vi "Settings Dialog.vi"(0 "Settings in":T9 {"Processing Settings"."Test Parameters"."Allowed Tolerance (%) FS" format="%#_4g"; "Acq Settings"."Config Settings"."Simulated Sensor Injection" scale=0.0..100.0}, 1 "Database in":refnum<queue>, 11 "error in (no error)":errorcluster) -> (3 "Database out":refnum<queue>, 4 "Settings out":T9 {"Processing Settings"."Test Parameters"."Allowed Tolerance (%) FS" format="%#_4g"; "Acq Settings"."Config Settings"."Simulated Sensor Injection" scale=0.0..100.0}, 6 "Measurements out":T7[](array[typedef]), 8 "UI Refresh Needed?":bool, 10 "Cancelled?":bool, 15 "error out":errorcluster)   [LabVIEW 2026, in "Settings.lvlib"]
doc: "Dialog for selecting user specified settings."
uses:
  Settings.lvlib
  controls/UI/Settings Cluster.ctl
  controls/UI/Acq Settings.ctl
  Acquisition/Instrument Specifications Configuration.ctl
  Acquisition/Instrument Specifications Cluster Configuration.ctl
  controls/UI/Measurement Role.ctl
  controls/UI/Config Settings.ctl
  Processing/Processing Settings.ctl
  controls/Messaging Payloads/Sensor CoreData.ctl
  controls/Messaging Payloads/Sensor CoreData Cluster.ctl
  controls/UI/Units Enum.ctl
  controls/UI/Signal Enum.ctl
  Processing/Test Parameters.ctl
  Processing/Test Parameters Cluster.ctl
  controls/UI/Test Sequence Context.ctl
  controls/UI/Direction.ctl
  controls/UI/Session Identfiers.ctl
  controls/UI/Test Sequence Settings.ctl
  controls/UI/Test Sequence State.ctl
  controls/UI/Test Sequence Enum.ctl
  controls/Controller/Stimulus Settings.ctl
  controls/Controller/Stimulus Outputs.ctl
  controls/Controller/Stimulus Output.ctl
  controls/Controller/Controller Core Data.ctl
  controls/Controller/Stimulus Output Configuration.ctl
  controls/Controller/Stimulus Role.ctl
  support/Architecture/Message Queue/Message Cluster.ctl
  controls/UI/Measurements Config.ctl
  controls/UI/Measurement Config.ctl
  controls/UI/Stimulus Outputs Display.ctl
  controls/UI/Stimulus Output Display.ctl
  controls/UI/Settings Refs.ctl
  controls/UI/UI List Type.ctl
  controls/UI/Data Entity.ctl
  controls/UI/Measurement Role Selection.ctl
  Acquisition/Acquisition.lvlib
  support/Architecture/Message Queue/Message Queue.lvlib
  Processing/Processing_Engine.lvlib
panel:
  in  "STIMULUS OUTPUTS":T1
  out "INSTRUMENT CONFIGURATIONS":T4
  in  "MEASUREMENTS":T8
  in  "Operator":string(combo)
  in  "Cancel Button":bool
  in  "OK Button":bool
  # "Non visible portion of dialog (needed for connector pane)."
  # "* Database-configured values. Maintained by an Administrator."
  # "Physical Channel and Measurement Role are assigned in the Measurements section."
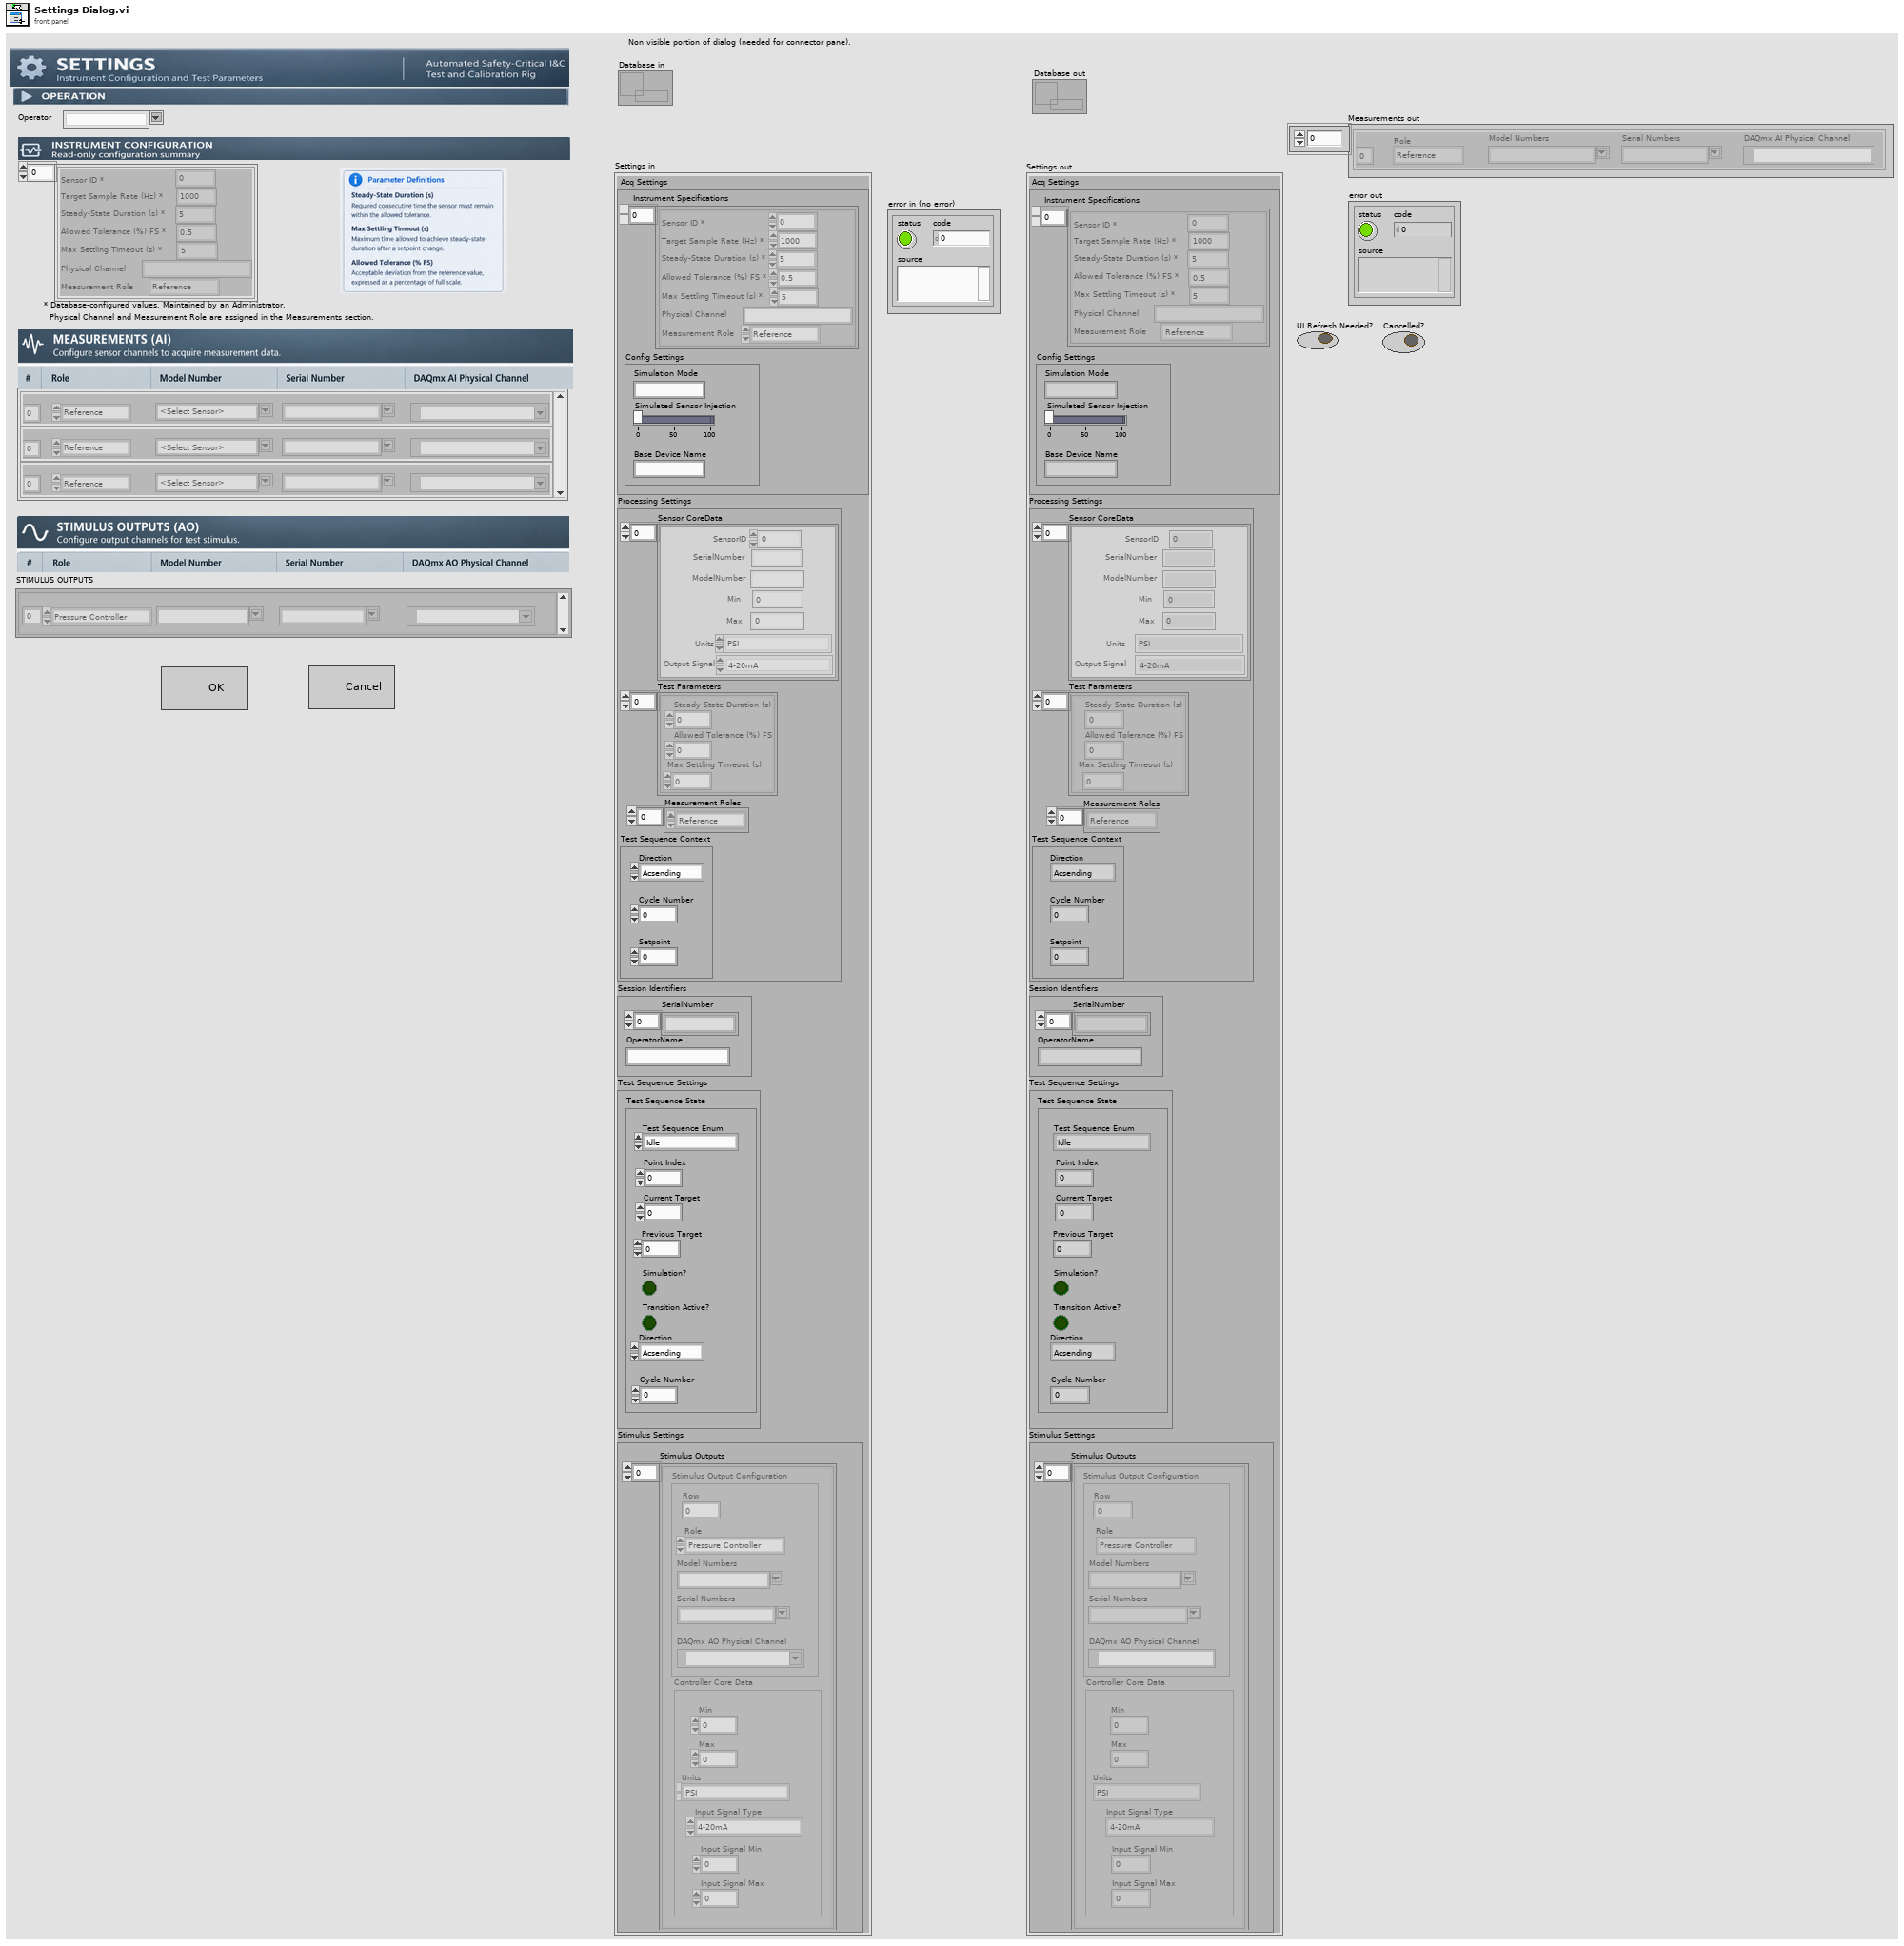
[diagram p1: front panel]
types:
  T1 = typedef "Settings.lvlib/Stimulus Outputs Display.ctl" = T2[]
  T2 = typedef "Settings.lvlib/Stimulus Output Display.ctl" = cluster{"DAQmx AO Physical Channel":tag, "Role":T3, "Model Numbers":string, "Serial Numbers":string, "Row":i32}
  T3 = typedef "Stimulus Role.ctl" = enum16{"Pressure Controller", "Temperature Controller"}
  T4 = typedef "Acquisition.lvlib/Instrument Specifications Configuration.ctl" = T5[]
  T5 = typedef "Acquisition.lvlib/Instrument Specifications Cluster Configuration.ctl" = cluster{"Sensor ID *":i32, "Target Sample Rate (Hz) *":dbl, "Steady-State Duration (s) *":i32, "Allowed Tolerance (%) FS *":dbl, "Max Settling Timeout (s) *":i32, "Physical Channel":string, "Measurement Role":T6}
  T6 = typedef "Settings.lvlib/Measurement Role.ctl" = enum16{"Reference", "UUT"}
  T7 = typedef "Measurement Config.ctl" = cluster{"DAQmx AI Physical Channel":tag, "Serial Numbers":string, "Model Numbers":string, "Role":T6, "Row":i32}
  T8 = typedef "Measurements Config.ctl" = T7[]
  T9 = typedef "Settings Cluster.ctl" = cluster{"Acq Settings":T10, "Processing Settings":T12, "Session Identifiers":T21, "Test Sequence Settings":T22, "Stimulus Settings":T25}
  T10 = typedef "Acq Settings.ctl" = cluster{"Instrument Specifications":T4, "Config Settings":T11}
  T11 = typedef "Config Settings.ctl" = cluster{"Simulated Sensor Injection":dbl, "Base Device Name":string, "Simulation Mode":string}
  T12 = typedef "Processing_Engine.lvlib/Processing Settings.ctl" = cluster{"Sensor CoreData":T13, "Test Parameters":T17, "Measurement Roles":T6[], "Test Sequence Context":T19}
  T13 = typedef "Sensor CoreData.ctl" = T14[]
  T14 = typedef "Settings.lvlib/Sensor CoreData Cluster.ctl" = cluster{"SerialNumber":string, "ModelNumber":string, "Min":dbl, "Max":dbl, "Units":T15, "Output Signal":T16, "SensorID":i32}
  T15 = typedef "Units Enum.ctl" = enum16{"PSI", "Deg C", "kPa", "GPM"}
  T16 = typedef "Signal Enum.ctl" = enum16{"4-20mA", "0-10V", "Thermocouple Type K"}
  T17 = typedef "Processing_Engine.lvlib/Test Parameters.ctl" = T18[]
  T18 = typedef "Settings.lvlib/Test Parameters Cluster.ctl" = cluster{"Steady-State Duration (s)":i32, "Allowed Tolerance (%) FS":dbl, "Max Settling Timeout (s)":i32}
  T19 = typedef "Settings.lvlib/Test Sequence Context.ctl" = cluster{"Direction":T20, "Cycle Number":i32, "Setpoint":dbl}
  T20 = typedef "Settings.lvlib/Direction.ctl" = enum16{"Acsending", "Descending"}
  T21 = typedef "Session Identfiers.ctl" = cluster{"SerialNumber":string[], "OperatorName":string}
  T22 = typedef "Test Sequence Settings.ctl" = cluster{"Test Sequence State":T23}
  T23 = typedef "Settings.lvlib/Test Sequence State.ctl" = cluster{"Test Sequence Enum":T24, "Point Index":i32, "Current Target":dbl, "Previous Target":dbl, "Simulation?":bool, "Direction":T20, "Transition Active?":bool, "Cycle Number":i32}
  T24 = typedef "Test Sequence Enum.ctl" = enum16{"Idle", "Start Point", "Point Complete", "Test Complete", "Abort Test", "Reset"}
  T25 = typedef "Settings.lvlib/Stimulus Settings.ctl" = cluster{"Stimulus Outputs":T26}
  T26 = typedef "Settings.lvlib/Stimulus Outputs.ctl" = T27[]
  T27 = typedef "Settings.lvlib/Stimulus Output.ctl" = cluster{"Controller Core Data":T28, "Stimulus Output Configuration":T29}
  T28 = typedef "Settings.lvlib/Controller Core Data.ctl" = cluster{"Min":dbl, "Max":dbl, "Units":T15, "Input Signal Type":T16, "Input Signal Min":dbl, "Input Signal Max":dbl}
  T29 = typedef "Settings.lvlib/Stimulus Output Configuration.ctl" = cluster{"DAQmx AO Physical Channel":tag, "Role":T3, "Model Numbers":string, "Serial Numbers":string, "Row":i32}
  T30 = typedef "Settings Refs.ctl" = cluster{"Serial Numbers Ref":refnum<vi>, "Logging Ref":refnum<vi>, "Model Numbers Ref":refnum<vi>, "OK Ref":refnum<vi>, "Instrument Specifications Cluster Ref":refnum<vi>, "Instrument Specifications Ref":refnum<vi>, "Measurements Ref":refnum<vi>, "Stimulus Outputs Ref":refnum<vi>}
  T31 = typedef "Settings.lvlib/Measurement Role Selection.ctl" = enum16{"Controller", "Reference", "UUT", "All"}
  T32 = typedef "Settings.lvlib/Data Entity.ctl" = enum16{"Measurement", "Controller", " Test Configuration"}
  T33 = enum8{"Enabled", "Disabled", "Disabled and Grayed Out"}
  T34 = typedef "UI List Type.ctl" = enum16{"Model Numbers", "Serial Numbers", "Operators", "Calibration Points", "Start Run Times"}
  T35 = typedef "LVPoint32TypeDef.ctl" = cluster{"Horizontal":i32, "Vertical":i32}
  T36 = typedef "MSG FetchConfiguration Payload.ctl" = cluster{"Serial Numbers":string[], "Hardware Settings Cluster":T5}
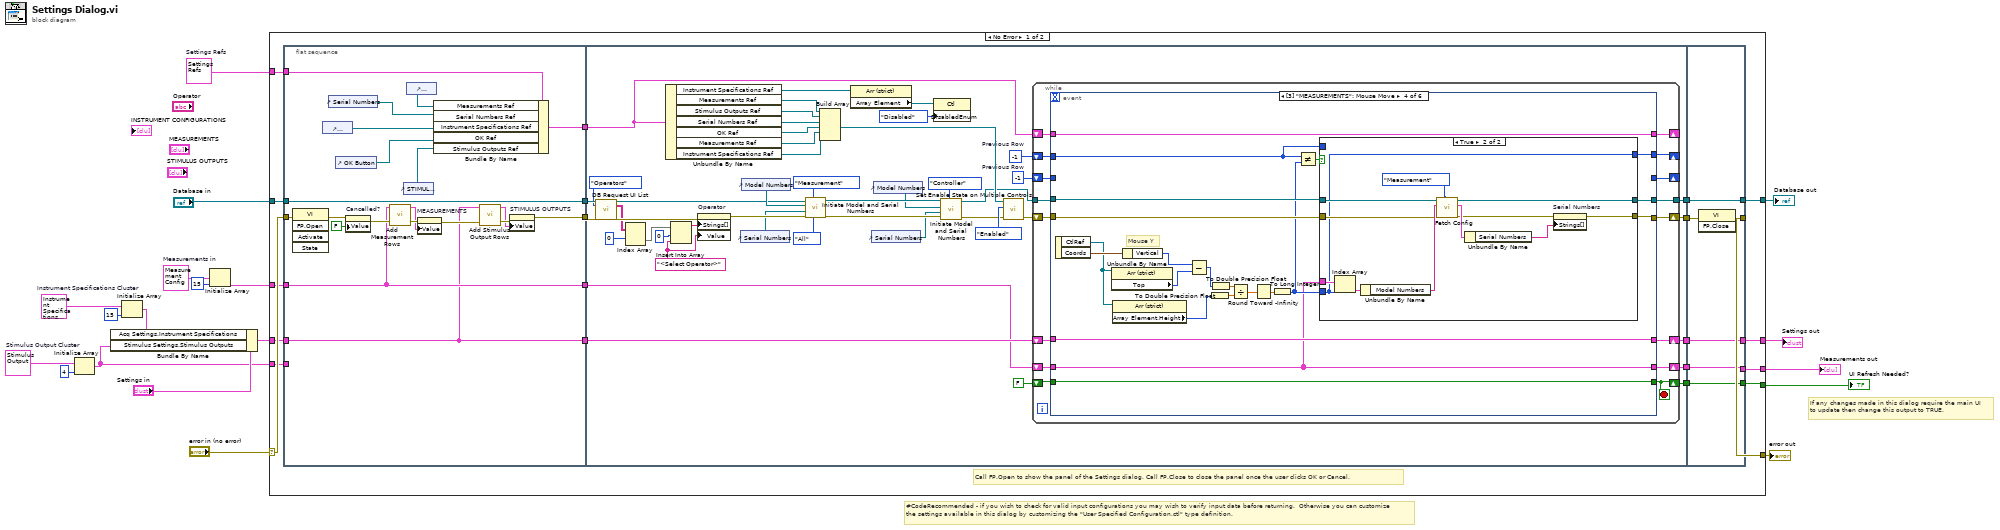
[diagram p0: block diagram]
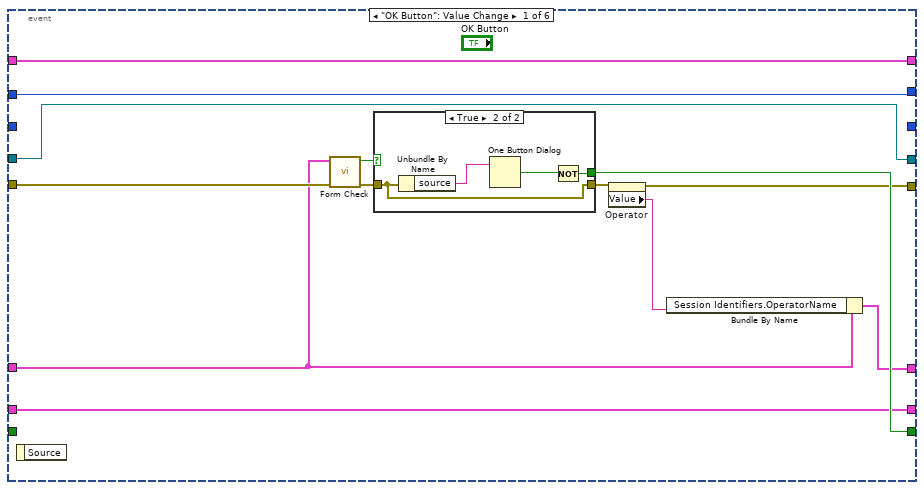
[diagram p2: hidden frame]
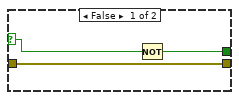
[diagram p3: hidden frame]
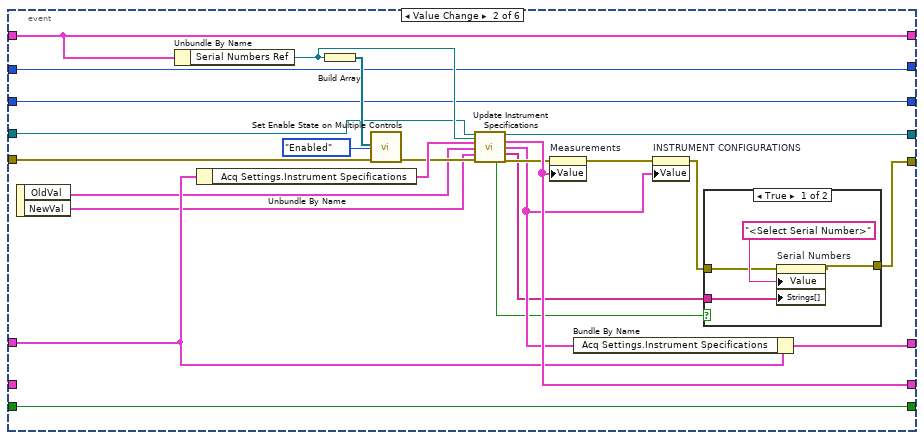
[diagram p4: hidden frame]
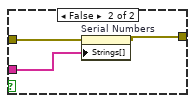
[diagram p5: hidden frame]
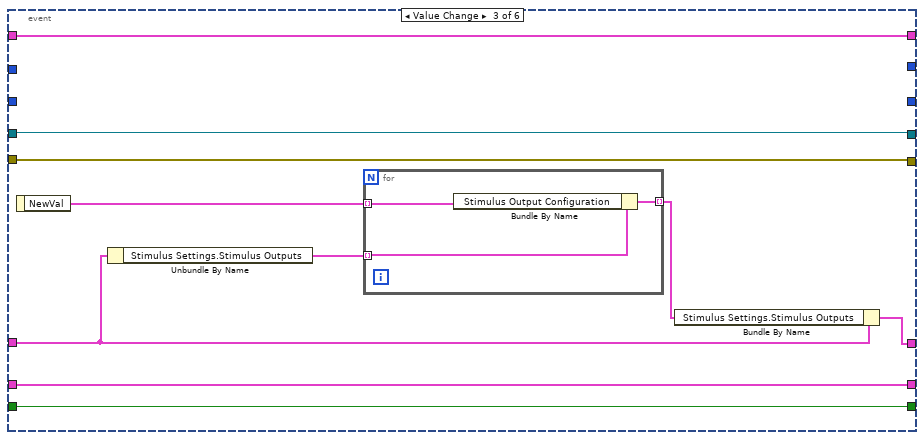
[diagram p6: hidden frame]
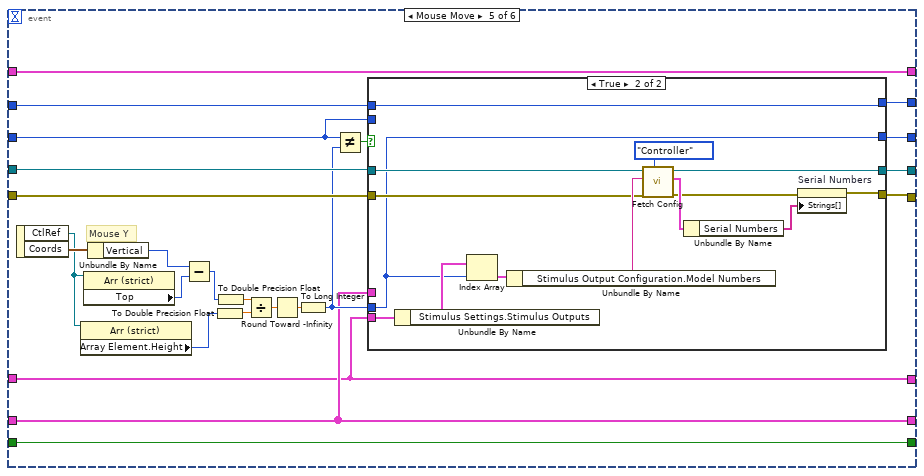
[diagram p8: hidden frame]
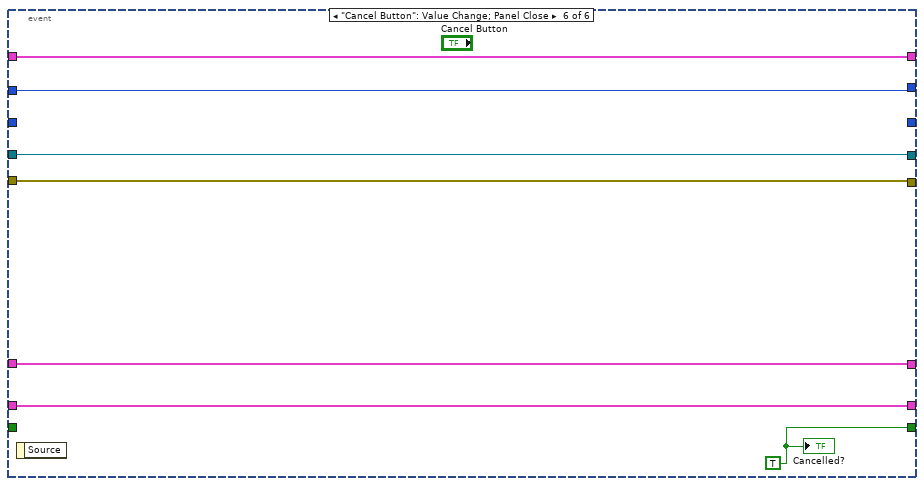
[diagram p10: hidden frame]
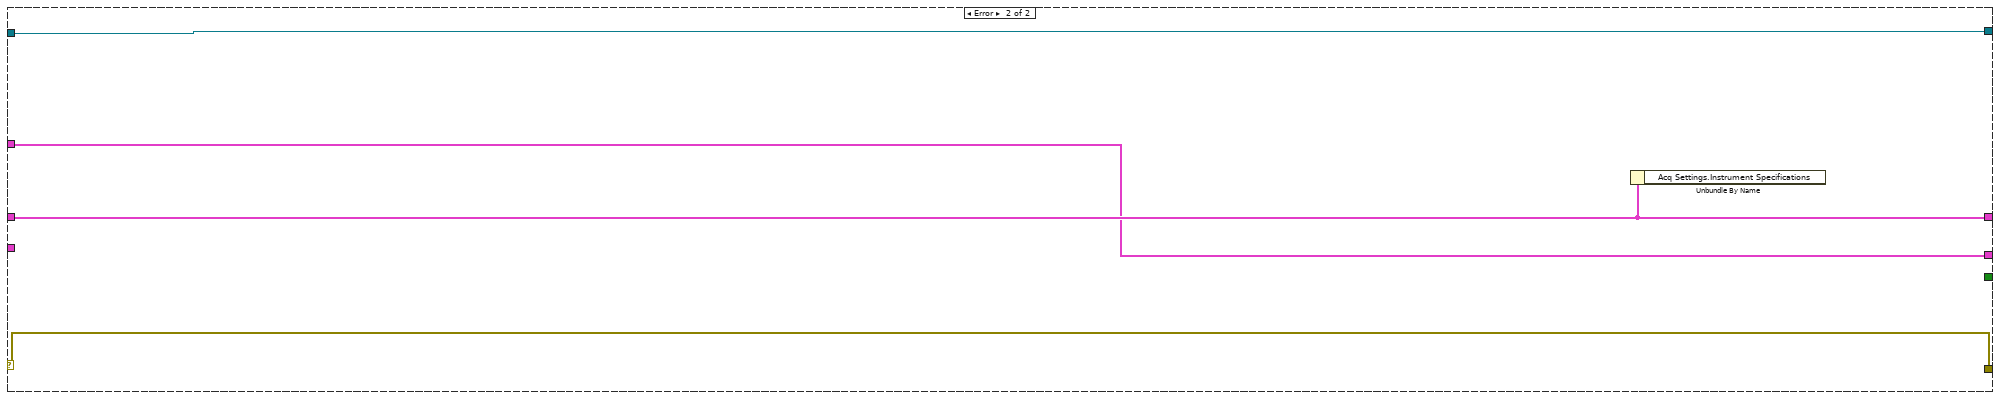
[diagram p11: hidden frame]
diagram:
  w2 = T27 {"Controller Core Data"={"Min"=0.0, "Max"=0.0, "Units"=enum."PSI", "Input Signal Type"=enum."4-20mA", "Input Signal Min"=0.0, "Input Signal Max"=0.0}, "Stimulus Output Configuration"={"DAQmx AO Physical Channel"="", "Role"=enum."Pressure Controller", "Model Numbers"="", "Serial Numbers"="", "Row"=0}}  # Stimulus Output Cluster
  w8 = T5 {"Sensor ID *"=0, "Target Sample Rate (Hz) *"=1000.0, "Steady-State Duration (s) *"=5, "Allowed Tolerance (%) FS *"=0.5, "Max Settling Timeout (s) *"=5, "Physical Channel"="", "Measurement Role"=enum."Reference"}  # Instrument Specifications Cluster
  w12 = T7 {"DAQmx AI Physical Channel"="", "Serial Numbers"="", "Model Numbers"="<Select Sensor>", "Role"=enum."Reference", "Row"=0}  # Measurements in
  w16 = T30 {"Serial Numbers Ref"=refnum, "Logging Ref"=refnum, "Model Numbers Ref"=refnum, "OK Ref"=refnum, "Instrument Specifications Cluster Ref"=refnum, "Instrument Specifications Ref"=refnum, "Measurements Ref"=refnum, "Stimulus Outputs Ref"=refnum}  # Settings Refs
  # "If any changes made in this dialog require the main UI to update then change this output to TRUE."
  # "#CodeRecommended - if you wish to check for valid input configurations you may wish to verify input data before returning.  Otherwise you can customize the settings available in this dialog by customizing the \"User Specified Configuration.ctl\" type definition."
  n1 = Initialize Array(w2, 4 ("dimension size")) -> (w1:T27[])
  n2 = Initialize Array(w8, 15 ("dimension size")) -> (w7:T5[])
  n3 = Bundle By Name(cluster="Settings in", "Acq Settings.Instrument Specifications"=w7, "Stimulus Settings.Stimulus Outputs"=w1) -> (w6:T9)
  n4 = Initialize Array(w12, 15 ("dimension size")) -> (w10:T7[])
  n5 = case shown="No Error" "error in (no error)" {
    selector: "error in (no error)" -> [w32 w282]
    tunnel: [w36 w282] -> w18
    tunnel: [w27 _] -> w17
    tunnel: "Database in" -> [w38 w280]
    tunnel: w16 -> [w33 _]
    tunnel: [w28 w281] -> w15
    tunnel: w6 -> [w30 w281]
    tunnel: [w25 w280] -> w14
    tunnel: w10 -> [w24 w279]
    tunnel: [w21 w279] -> w13
    tunnel: w1 -> [w20 _]
    frame No Error {
      # "Call FP.Open to show the panel of the Settings dialog. Call FP.Close to close the panel once the user clicks OK or Cancel."
      n6 = flat-sequence {
        tunnel: w38 -> [w59]
        tunnel: [w44] -> w35
        tunnel: w32 -> [w60]
        tunnel: [w59] -> w34
        tunnel: w33 -> [w56]
        tunnel: [w58] -> w31
        tunnel: w30 -> [w41]
        tunnel: [w41] -> w29
        tunnel: w24 -> [w42]
        tunnel: [w42] -> w23
        tunnel: w20 -> [_]
        tunnel: [w106] -> w40
        tunnel: [w105] -> w39
        tunnel: w35 -> [w98]
        tunnel: [w104] -> w37
        tunnel: w34 -> [w99]
        tunnel: w31 -> [w101]
        tunnel: w29 -> [w100]
        tunnel: [w92] -> w26
        tunnel: w23 -> [w88]
        tunnel: [w91] -> w22
        tunnel: [w278] -> w28
        tunnel: w40 -> [w275]
        tunnel: w39 -> [w278]
        tunnel: w37 -> [w277]
        tunnel: [w276] -> w36
        tunnel: [w275] -> w27
        tunnel: w26 -> [w274]
        tunnel: [w274] -> w25
        tunnel: w22 -> [w273]
        tunnel: [w273] -> w21
        frame #0 {
          n7 = invoke class="VI" method="FP.Open"(error in=w60) -> (error out=w55:errorcluster)  [unwired: 4 in, 4 out]
          n8 = control-ref of="INSTRUMENT CONFIGURATIONS"() -> (w50:refnum<vi>)
          n9 = control-ref of="Serial Numbers"() -> (w53:refnum<vi>)
          n10 = control-ref of="OK Button"() -> (w57:refnum<vi>)
          n11 = property on="Cancelled?" class="Bool (strict)"(error in=w55, "Value"=FALSE ("Cancelled?")) -> (error out=w49:errorcluster)  [unwired: 1 in, 1 out]
          n12 = call "Add Measurement Rows.vi"("error in (no error)"=w49, "Measurements in"=w42) -> ("error out"=w48:errorcluster, "Measurements out"=w47:T8)  [unwired: 8 in]
          n13 = control-ref of="STIMULUS OUTPUTS"() -> (w51:refnum<vi>)
          n14 = control-ref of="MEASUREMENTS"() -> (w52:refnum<vi>)
          n15 = property on="MEASUREMENTS" class="Arr (strict)"(error in=w48, "Value"=w47) -> (error out=w46:errorcluster)  [unwired: 1 in, 1 out]
          n16 = Bundle By Name(cluster=w56, "Measurements Ref"=w52, "Serial Numbers Ref"=w53, "Instrument Specifications Ref"=w50, "OK Ref"=w57, "Stimulus Outputs Ref"=w51) -> (w58:T30)
          n17 = call "Add Stimulus Output Rows.vi"("error in (no error)"=w46, "Settings"=w41) -> ("error out"=w45:errorcluster, "Stimulus Outputs"=w43:T1)  [unwired: 8 in]
          n18 = property on="STIMULUS OUTPUTS" class="Arr (strict)"(error in=w45, "Value"=w43) -> (error out=w44:errorcluster)  [unwired: 1 in, 1 out]
        }
        frame #1 {
          w65 = -1  # Previous Row
          w89 = -1  # Previous Row
          w93 = "<Select Operator>"
          n19 = call "DB Request UI List.vi"("Database in"=w99, "UI List Type"=UI_List_Type."Operators", "error in (no error)"=w98) -> ("Database out"=w75:refnum<queue>, "Results"=w64:string[][], "error out"=w95:errorcluster)  [unwired: 14 in]
          n20 = Index Array(array=w64, index (row)=0 ("index")) -> (element=w62:string[])  [unwired: 1 in]
          n21 = Unbundle By Name(w101) -> ("Instrument Specifications Ref"=w80:refnum<vi>, "Measurements Ref"=w84:refnum<vi>, "Stimulus Outputs Ref"=w86:refnum<vi>, "Serial Numbers Ref"=w85:refnum<vi>, "OK Ref"=w82:refnum<vi>, "Measurements Ref"=w83:refnum<vi>, "Instrument Specifications Ref"=w81:refnum<vi>)
          n22 = Insert Into Array(array=w62, index=0, new element=w93) -> (w96:string[])
          n23 = property on="Operator" class="CmbBox"(error in=w95, "Strings[]"=w96, "Value"=w93) -> (error out=w94:errorcluster)  [unwired: 1 in, 1 out]
          n24 = control-ref of="Serial Numbers"() -> (w74:refnum<vi>)
          n25 = control-ref of="Model Numbers"() -> (w76:refnum<vi>)
          n26 = call "Initiate Model and Serial Numbers.vi"("Measurement Role Selection"=Measurement_Role_Selection."All" ("Measurement Role"), "UI Device Type"=Data_Entity."Measurement", "error in (no error)"=w94, "Serial CmbBox Ref"=w74, "Model CmbBox Ref"=w76, "Database in"=w75) -> ("error out"=w73:errorcluster, "Database out"=w71:refnum<queue>)  [unwired: 4 in]
          n27 = Build Array(w84, w86, w85, w82, w83, w81) -> (w102:refnum<vi>[])
          n28 = property class="Arr (strict)"(reference=w80) -> ("Array Element"=w79:refnum<vi>)  [unwired: 1 in, 2 out]
          n29 = control-ref of="Serial Numbers"() -> (w66:refnum<vi>)
          n30 = control-ref of="Model Numbers"() -> (w67:refnum<vi>)
          n31 = property class="Ctl"(reference=w79, "DisabledEnum"=T33."Disabled" ("Disabled")) -> ()  [unwired: 1 in, 2 out]
          n32 = call "Initiate Model and Serial Numbers.vi"("UI Device Type"=Data_Entity."Controller", "error in (no error)"=w73, "Serial CmbBox Ref"=w66, "Model CmbBox Ref"=w67, "Database in"=w71) -> ("error out"=w72:errorcluster, "Database out"=w70:refnum<queue>)  [unwired: 5 in]
          n33 = call "Set Enable State on Multiple Controls.vi"("Controls"=w102, "Disabled"=T33."Enabled", "error in (no error)"=w72) -> ("error out"=w77:errorcluster)  [unwired: 7 in]
          n34 = while {
            tunnel: w70 -> [w118]
            shift-right: [w122] -> w105
            shift-left: w100 -> [w121]
            shift-right: [w120] -> w104
            shift-left: w77 -> [w119]
            shift-right: [w114] -> w106
            shift-left: FALSE ("UI Refresh Needed?") -> [w117]
            shift-right: [w115] -> _
            shift-left: w101 -> [w116]
            tunnel: [w113] -> w92
            shift-right: [w109] -> _
            shift-left: w89 -> [w110]
            shift-right: [w112] -> w91
            shift-left: w88 -> [w111]
            shift-right: [w107] -> _
            shift-left: w65 -> [w108]
            stop <- w114 stop-if-true
            n35 = event shown="[3] \"MEASUREMENTS\": Mouse Move" {
              selector: _ -> [_ _ _ _ _ _]
              dyn-events: _ -> [_ _ _ _ _ _]
              timeout: _ -> [_ _ _ _ _ _]
              tunnel: [w128 w160 w178 w208 w225 w272] -> w122
              tunnel: w121 -> [w125 w161 w180 w208 w225 w272]
              tunnel: [w132 w166 w176 w187 w228 w270] -> w114
              tunnel: w119 -> [w134 w159 w175 w195 w235 w271]
              tunnel: [w126 w150 w175 w189 w230 w271] -> w120
              tunnel: w118 -> [w127 w145 w182 w196 w236 w268]
              tunnel: w117 -> [_ w166 w176 w187 w228 _]
              tunnel: w116 -> [w131 w147 w183 w207 w247 w269]
              tunnel: [w131 w147 w183 w207 w247 w269] -> w115
              tunnel: [w127 w144 w182 w194 w234 w268] -> w113
              tunnel: [w124 w165 w177 w188 w229 w267] -> w112
              tunnel: w111 -> [w124 _ w177 w188 w229 w267]
              tunnel: w110 -> [w123 w148 _ w190 w231 w266]
              tunnel: [w123 w148 _ w191 w232 w266] -> w109
              tunnel: w108 -> [_ w143 _ _ w226 _]
              tunnel: [_ w143 _ _ w224 _] -> w107
              event "OK Button": Value Change {
                n36 = event-data() -> ()  [unwired: 1 in, 1 out]
                n37 = call "Form Check.vi"("error in (no error)"=w134, "Config in"=w125) -> ("error out"=w133:errorcluster, "Form Error?"=w135:bool)  [unwired: 8 in]
                n38 = case shown="True" w135 {
                  selector: w135 -> [w137 _]
                  tunnel: w133 -> [w136 w139]
                  tunnel: [w138 w140] -> w132
                  tunnel: [w136 w139] -> w130
                  frame False {
                    n39 = Not(x=w137) -> (.not. x?=w138:bool)
                  }
                  frame True {
                    n40 = Unbundle By Name(w139) -> ("source"=w142:string)
                    n41 = One Button Dialog(message=w142) -> (true=w141:bool)  [unwired: 1 in]
                    n42 = Not(x=w141) -> (.not. x?=w140:bool)
                  }
                }
                n43 = property on="Operator" class="CmbBox"(error in=w130) -> (error out=w126:errorcluster, "Value"=w129:string)  [unwired: 1 in, 1 out]
                n44 = Bundle By Name(cluster=w125, "Session Identifiers.OperatorName"=w129) -> (w128:T9)
              }
              event Value Change {
                n45 = event-data() -> ("OldVal"=w157:T8, "NewVal"=w156:T8)  [unwired: 1 in]
                n46 = Unbundle By Name(w147) -> ("Serial Numbers Ref"=w155:refnum<vi>)
                n47 = Unbundle By Name(w161) -> ("Acq Settings.Instrument Specifications"=w162:T4)
                n48 = Build Array(w155) -> (w154:refnum<vi>[])
                n49 = call "Set Enable State on Multiple Controls.vi"("Controls"=w154, "Disabled"=T33."Enabled", "error in (no error)"=w159) -> ("error out"=w158:errorcluster)  [unwired: 7 in]
                n50 = call "Update Instrument Specifications.vi"("Queue in"=w145, "Serial Numbers Ref"=w155, "Instrument Specifications in"=w162, "OldVal"=w157, "NewVal"=w156, "error in (no error)"=w158) -> ("Queue out"=w144:refnum<queue>, "Measurements"=w165:T7[], "Instrument Specifications out"=w153:T4, "Serial Numbers"=w149:string[], "Serial Number Header?"=w152:bool, "error out"=w164:errorcluster)  [unwired: 4 in]
                n51 = property on="Measurements" class="Arr (strict)"(error in=w164, "Value"=w165) -> (error out=w163:errorcluster)  [unwired: 1 in, 1 out]
                n52 = Bundle By Name(cluster=w161, "Acq Settings.Instrument Specifications"=w153) -> (w160:T9)
                n53 = property on="INSTRUMENT CONFIGURATIONS" class="Arr (strict)"(error in=w163, "Value"=w153) -> (error out=w151:errorcluster)  [unwired: 1 in, 1 out]
                n54 = case shown="True" w152 {
                  tunnel: w151 -> [w169 w173]
                  tunnel: [w168 w172] -> w150
                  tunnel: w149 -> [w167 w171]
                  frame True {
                    n55 = property on="Serial Numbers" class="CmbBox"(error in=w169, "Value"="<Select Serial Number>", "Strings[]"=w167) -> (error out=w168:errorcluster)  [unwired: 1 in, 1 out]
                  }
                  frame False {
                    n56 = property on="Serial Numbers" class="CmbBox"(error in=w173, "Strings[]"=w171) -> (error out=w172:errorcluster)  [unwired: 1 in, 1 out]
                  }
                }
              }
              event Value Change {
                n57 = event-data() -> ("NewVal"=w174:T1)  [unwired: 1 in]
                n58 = Unbundle By Name(w180) -> ("Stimulus Settings.Stimulus Outputs"=w181:T26)
                n59 = for {
                  tunnel: w181 -> [w186] mode=indexing
                  tunnel: w174 -> [w184] mode=indexing
                  tunnel: [w185] -> w179 mode=indexing
                  n60 = Bundle By Name(cluster=w186, "Stimulus Output Configuration"=w184) -> (w185:T27)
                }
                n61 = Bundle By Name(cluster=w180, "Stimulus Settings.Stimulus Outputs"=w179) -> (w178:T9)
              }
              event Mouse Move {
                # "Mouse Y"
                n62 = event-data() -> ("CtlRef"=w203:refnum<vi>, "Coords"=w206:T35)  [unwired: 1 in]
                n63 = property class="Arr (strict)"(reference=w203) -> ("Top"=w204:i32)  [unwired: 1 in, 2 out]
                n64 = property class="Arr (strict)"(reference=w203) -> ("Array Element.Height"=w200:u32)  [unwired: 1 in, 2 out]
                n65 = Unbundle By Name(w206) -> ("Vertical"=w205:i32)
                n66 = Subtract(x=w205, y=w204) -> (x-y=w202:i32)
                n67 = To Double Precision Float(number=w200) -> (double precision float=w199:dbl)
                n68 = To Double Precision Float(number=w202) -> (double precision float=w201:dbl)
                n69 = Divide(x=w201, y=w199) -> (x/y=w198:dbl)
                n70 = Round Toward -Infinity(1:w198) -> (0:w197:dbl)
                n71 = To Long Integer(number=w197) -> (32bit integer=w193:i32)
                n72 = Not Equal?(x=w190, y=w193) -> (x != y?=w192:bool)
                n73 = case shown="True" w192 {
                  tunnel: w188 -> [_ w223]
                  tunnel: w196 -> [w210 w220]
                  tunnel: w195 -> [w209 w219]
                  tunnel: [w210 w218] -> w194
                  tunnel: [w209 w214] -> w189
                  tunnel: w193 -> [_ w216]
                  tunnel: [w211 w216] -> w191
                  tunnel: w190 -> [w211 _]
                  frame False {
                  }
                  frame True {
                    n74 = Index Array(array=w223, index=w216) -> (element=w222:T7)
                    n75 = Unbundle By Name(w222) -> ("Model Numbers"=w221:string)
                    n76 = call "Fetch Config.vi"("UI Device Type"=Data_Entity."Measurement", "error in (no error)"=w219, "ModelNumber"=w221, "Database in"=w220) -> ("error out"=w215:errorcluster, "Model Details Payload"=w217:T36, "Database out"=w218:refnum<queue>)  [unwired: 5 in]
                    n77 = Unbundle By Name(w217) -> ("Serial Numbers"=w213:string[])
                    n78 = property on="Serial Numbers" class="CmbBox"(error in=w215, "Strings[]"=w213) -> (error out=w214:errorcluster)  [unwired: 1 in, 1 out]
                  }
                }
              }
              event Mouse Move {
                # "Mouse Y"
                n79 = event-data() -> ("CtlRef"=w243:refnum<vi>, "Coords"=w246:T35)  [unwired: 1 in]
                n80 = property class="Arr (strict)"(reference=w243) -> ("Array Element.Height"=w240:u32)  [unwired: 1 in, 2 out]
                n81 = property class="Arr (strict)"(reference=w243) -> ("Top"=w244:i32)  [unwired: 1 in, 2 out]
                n82 = Unbundle By Name(w246) -> ("Vertical"=w245:i32)
                n83 = Subtract(x=w245, y=w244) -> (x-y=w242:i32)
                n84 = To Double Precision Float(number=w240) -> (double precision float=w239:dbl)
                n85 = To Double Precision Float(number=w242) -> (double precision float=w241:dbl)
                n86 = Divide(x=w241, y=w239) -> (x/y=w238:dbl)
                n87 = Round Toward -Infinity(1:w238) -> (0:w237:dbl)
                n88 = To Long Integer(number=w237) -> (32bit integer=w233:i32)
                n89 = Not Equal?(x=w226, y=w233) -> (x != y?=w227:bool)
                n90 = case shown="True" w227 {
                  tunnel: w229 -> [_ _]
                  tunnel: w236 -> [w250 w264]
                  tunnel: w235 -> [w249 w263]
                  tunnel: [w250 w262] -> w234
                  tunnel: [w249 w253] -> w230
                  tunnel: w233 -> [_ w256]
                  tunnel: [w251 w255] -> w232
                  tunnel: w231 -> [w251 w255]
                  tunnel: w226 -> [w248 _]
                  tunnel: w225 -> [_ w259]
                  tunnel: [w248 w256] -> w224
                  frame False {
                  }
                  frame True {
                    n91 = Unbundle By Name(w259) -> ("Stimulus Settings.Stimulus Outputs"=w258:T26)
                    n92 = Index Array(array=w258, index=w256) -> (element=w257:T27)
                    n93 = Unbundle By Name(w257) -> ("Stimulus Output Configuration.Model Numbers"=w265:string)
                    n94 = call "Fetch Config.vi"("UI Device Type"=Data_Entity."Controller", "error in (no error)"=w263, "ModelNumber"=w265, "Database in"=w264) -> ("error out"=w254:errorcluster, "Model Details Payload"=w261:T36, "Database out"=w262:refnum<queue>)  [unwired: 5 in]
                    n95 = Unbundle By Name(w261) -> ("Serial Numbers"=w252:string[])
                    n96 = property on="Serial Numbers" class="CmbBox"(error in=w254, "Strings[]"=w252) -> (error out=w253:errorcluster)  [unwired: 1 in, 1 out]
                  }
                }
              }
              event "Cancel Button": Value Change; Panel Close {
                w270 = TRUE ("UI Refresh Needed?")
                n97 = event-data() -> ()  [unwired: 1 in, 1 out]
                "Cancelled?" <- w270
              }
            }
          }
        }
        frame #2 {
          n98 = invoke class="VI" method="FP.Close"(error in=w277) -> (error out=w276:errorcluster)  [unwired: 2 in, 2 out]
        }
      }
    }
    frame Error {
      n99 = Unbundle By Name(w281) -> ()  [unwired: 1 out]
    }
  }
  "UI Refresh Needed?" <- w17
  "error out" <- w18
  "Settings out" <- w15
  "Database out" <- w14
  "Measurements out" <- w13
